vi "SaveGeorgePrefs.vi"(7 "GlobalPrefs":path, 10 "plots":refnum<vi>[](array[refnum]), 11 "Test Name":string) -> (0 "error out":errorcluster, 2 "Settings":T2)   [LabVIEW 2022 SP3]
uses:
  <vilib>/Utility/miscctls.llb/LVRangeTypeDef.ctl
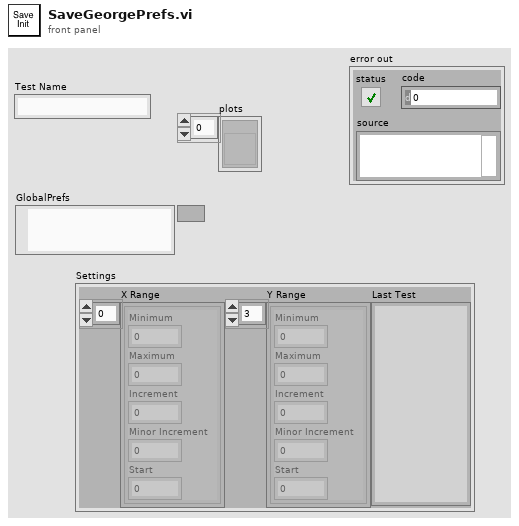
[diagram p1: front panel]
types:
  T1 = typedef "LVRangeTypeDef.ctl" = cluster{"Minimum":dbl, "Maximum":dbl, "Increment":dbl, "Minor Increment":dbl, "Start":dbl}
  T2 = cluster{"X Range":T1[], "Y Range":T1[], "Last Test":string}
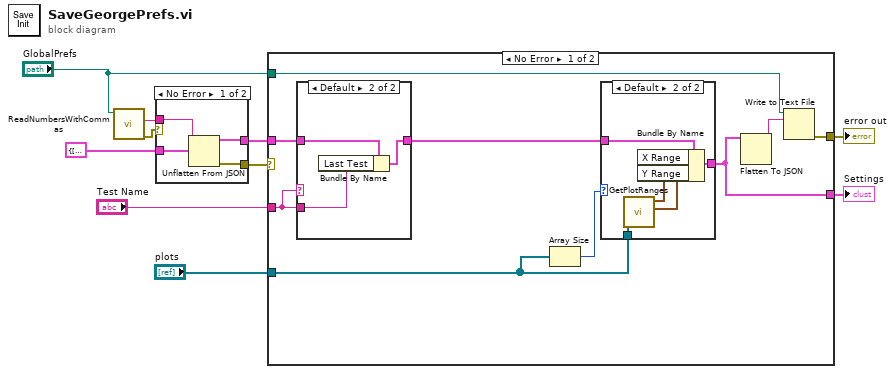
[diagram p0: block diagram]
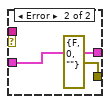
[diagram p2: hidden frame]
diagram:
  n1 = call "ReadNumbersWithCommas.vi"("file (use dialog)"="GlobalPrefs") -> ("error out"=w3:errorcluster, "text"=w2:string)  [unwired: 7 in, 2 out]
  n2 = case shown="No Error" w3 {
    tunnel: w2 -> [w14 _]
    tunnel: T2 {"X Range"=[{"Minimum"=200.0, "Maximum"=10000.0, "Increment"=2500.0, "Minor Increment"=500.0, "Start"=2500.0}, {"Minimum"=0.0, "Maximum"=0.05, "Increment"=0.025, "Minor Increment"=0.0025, "Start"=0.0}, {"Minimum"=0.0, "Maximum"=0.3, "Increment"=0.1, "Minor Increment"=0.01, "Start"=0.0}, {"Minimum"=200.0, "Maximum"=10000.0, "Increment"=10.0, "Minor Increment"=100.0, "Start"=1000.0}], "Y Range"=[{"Minimum"=-25.0, "Maximum"=0.0, "Increment"=5.0, "Minor Increment"=1.0, "Start"=-25.0}, {"Minimum"=-100.0, "Maximum"=100.0, "Increment"=50.0, "Minor Increment"=10.0, "Start"=-100.0}, {"Minimum"=-100.0, "Maximum"=100.0, "Increment"=50.0, "Minor Increment"=10.0, "Start"=-100.0}, {"Minimum"=-30.0, "Maximum"=30.0, "Increment"=5.0, "Minor Increment"=1.0, "Start"=-30.0}], "Last Test"="ScratchPad"} ("Default") -> [w13 w16]
    tunnel: [w12 errorcluster {"status"=FALSE, "code"=0, "source"=""} ("error out")] -> w9
    tunnel: [w11 w16] -> w8
    frame No Error {
      n3 = Unflatten From JSON(JSON string=w14, type and defaults=w13) -> (value=w11:T2, error out=w12:errorcluster)  [unwired: 5 in]
    }
    frame Error {
    }
  }
  n4 = case shown="No Error" w9 {
    tunnel: w8 -> [w25 w36]
    tunnel: "Test Name" -> [w23 _]
    tunnel: [w21 w36] -> w6
    tunnel: "GlobalPrefs" -> [w22 _]
    tunnel: "plots" -> [w19 _]
    tunnel: [w18 _] -> w4
    frame No Error {
      n5 = case shown="Default" w23 {
        tunnel: w25 -> [w32 w35]
        tunnel: w23 -> [_ w34]
        tunnel: [w32 w33] -> w17
        frame "" {
        }
        frame Default {
          n6 = Bundle By Name(cluster=w35, "Last Test"=w34) -> (w33:T2)
        }
      }
      n7 = Array Size(array=w19) -> (size(s)=w20:i32)
      n8 = case shown="Default" w20 {
        tunnel: w17 -> [w26 w31]
        tunnel: [w26 w30] -> w21
        tunnel: w19 -> [_ w29]
        frame 0 {
        }
        frame Default {
          n9 = call "GetPlotRanges.vi"("plots"=w29) -> ("Yscales"=w27:T1[], "Xscales"=w28:T1[])  [unwired: 9 in]
          n10 = Bundle By Name(cluster=w31, "X Range"=w28, "Y Range"=w27) -> (w30:T2)
        }
      }
      n11 = Flatten To JSON(anything=w21) -> (JSON string=w24:string)  [unwired: 2 in, 1 out]
      n12 = Write to Text File(file (use dialog)=w22, text=w24) -> (error out=w18:errorcluster)  [unwired: 2 in, 2 out]
    }
    frame Error {
    }
  }
  "Settings" <- w6
  "error out" <- w4
